vi "Tenerowicz_10_target_1.vi"   [LabVIEW 2020]
uses:
  <vilib>/Platform/TimedLoop/XDataNode/timing_clust.ctl
  <vilib>/Platform/TimedLoop/XDataNode/nitl_modes.ctl
  <vilib>/Platform/TimedLoop/XDataNode/wakeup.ctl
  <vilib>/platform/TimedLoop/XDataNode/XDataNode.xnode
  <vilib>/Platform/TimedLoop/XDataNode/XDNodeRunTimeDep.lvlib
types:
  T1 = typedef "XDNodeRunTimeDep.lvlib/timing_clust.ctl" = cluster{"Expected End [f-1]":u64, "Actual End [f-1]":u64, "Finished Late? [f-1]":bool, "Expected End [i-1]":u64, "Actual End [i-1]":u64, "Finished Late? [i-1]":bool, "Expected Start [i]":u64, "Actual Start [i]":u64, "Expected Start [f]":u64, "Actual Start [f]":u64, "Source Name":string, "Structure Name":string, "Period":i64, "Deadline":i64, "Offset":i64, "Start":i64, "Priority":i32, "Timeout":i32, "Mode":T2, "Wakeup Reason":T3, "Error":errorcluster, "Source Type":string, "Secondary Source Type":string, "Global End Time":u64, "Global Start Time":u64, "Frame Duration":u64, "Iteration Duration":u64, "Assigned CPU":i32, "I/O Scan Engine Mode":u32}
  T2 = typedef "XDNodeRunTimeDep.lvlib/nitl_modes.ctl" = enum32{"No Change", "Process missed periods, maintain original phase", "Discard missed periods, maintain original phase", "Process missed periods, ignore original phase", "Discard missed periods, ignore original phase"}
  T3 = typedef "XDNodeRunTimeDep.lvlib/wakeup.ctl" = enum32{"Normal", "Aborted", "Asynchronous wakeup", "Timing source error", "Timed loop error", "Timeout"}
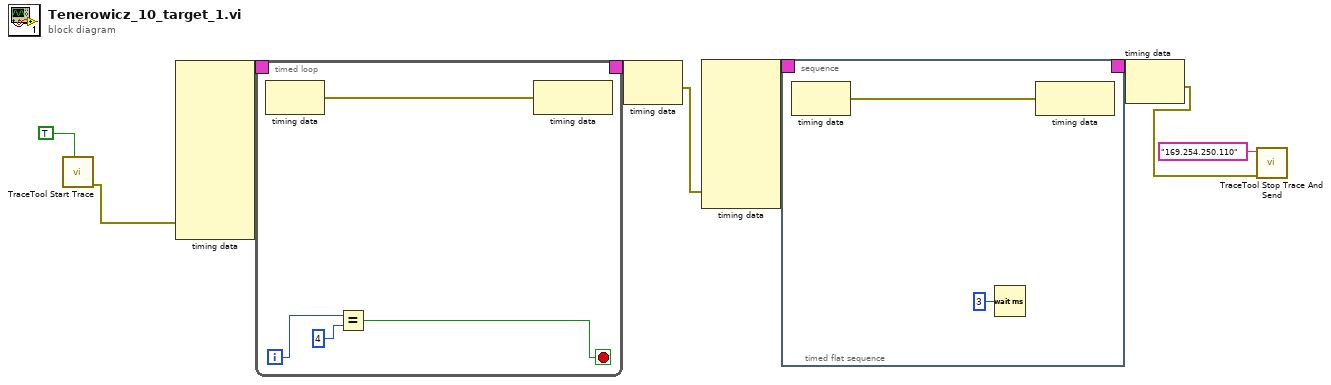
[diagram p0: block diagram]
diagram:
  n1 = call <vilib>:"TraceTool Start Trace.vi"("Detailed Tracing? (F)"=TRUE) -> ("error out"=w3:errorcluster)  [unwired: 9 in, 1 out]
  n2 = node-c288(w3) -> (w9:T1)  [unwired: 9 in]
  n3 = timed-loop {
    timing: w9 -> [_]
    timing-out: [_] -> w8
    i -> [w12]
    stop <- w10 stop-if-true
    n4 = node-c288() -> (w13:errorcluster)  [unwired: 1 in]
    n5 = Equal?(x=w12, y=4) -> (x = y?=w10:bool)
    n6 = node-c288(w13) -> ()  [unwired: 1 out]
  }
  n7 = node-c288(w8) -> (w1:errorcluster)
  n8 = node-c288(w1) -> (w7:T1)  [unwired: 7 in]
  n9 = timed-sequence {
    timing: w7 -> [_]
    timing-out: [_] -> w6
    n10 = timed-flat-sequence {
      n11 = node-c288() -> (w19:errorcluster)  [unwired: 1 in]
      n12 = Wait (ms)(milliseconds to wait=u32 3) -> ()  [unwired: 1 out]
      n13 = node-c288(w19) -> ()  [unwired: 1 out]
    }
  }
  n14 = node-c288(w6) -> (w2:errorcluster)
  n15 = call <vilib>:"TraceTool Stop Trace And Send.vi"("error in (no error)"=w2, "Trace Host Network Address"="169.254.250.110") -> ()  [unwired: 9 in, 1 out]
